vi "getClientID.vi"(11 "CONNECT in":refnum<class "CONNECT.lvclass">) -> (2 "Client ID":string, 3 "CONNECT out":refnum<class "CONNECT.lvclass">)   [LabVIEW 2013, in "CONNECT.lvclass"]
uses:
  CONNECT.lvclass
  ControlPacket/ControlPacket.lvclass/ControlPacket.ctl
  ControlPacket/ControlPacket.lvclass
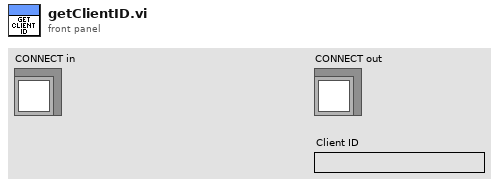
[diagram p1: front panel]
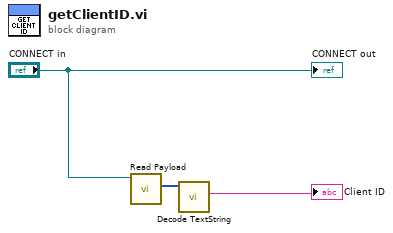
[diagram p0: block diagram]
diagram:
  n1 = call "Read Payload.vi"("ControlPacket in"="CONNECT in") -> ("Payload"=w3:u8[])  [unwired: 9 in, 1 out]
  n2 = call "Decode TextString.vi"("Length-Prefixed Field"=w3) -> ("Text String"=→"Client ID":string)  [unwired: 9 in, 1 out]
  "CONNECT out" <- "CONNECT in"
